vi "Framework Configuration.Get All Transfer Configurations.vi"(8 "error in (no error)":errorcluster, 11 "Framework Configuration in":refnum<class "Framework Configuration.lvclass">) -> (0 "error out":errorcluster, 2 "Transfer Configurations":T1[](array[typedef]), 3 "Framework Configuration out":refnum<class "Framework Configuration.lvclass">)   [LabVIEW 2017, in "DSF.Engine.lvlib" / "Framework Configuration.lvclass"]
uses:
  Framework Configuration.lvclass
  DSF Configuration API/1.0.0/Public/Controls/DSF Engine Transfer Configuration.ctl
  DSF Configuration API/1.0.0/Public/Controls/DSF Byte Order.ctl
  DSF Configuration API/1.0.0/Public/Controls/DSF Engine Channel Configuration.ctl
  DSF Configuration API/1.0.0/Public/Controls/DSF Data Type.ctl
  DSF Configuration API/1.0.0/Public/Controls/DSF Settings Info.ctl
  Framework Configuration.lvclass/Framework Configuration.ctl
  DSF Configuration API/1.0.0/DSF Configuration API.lvlib
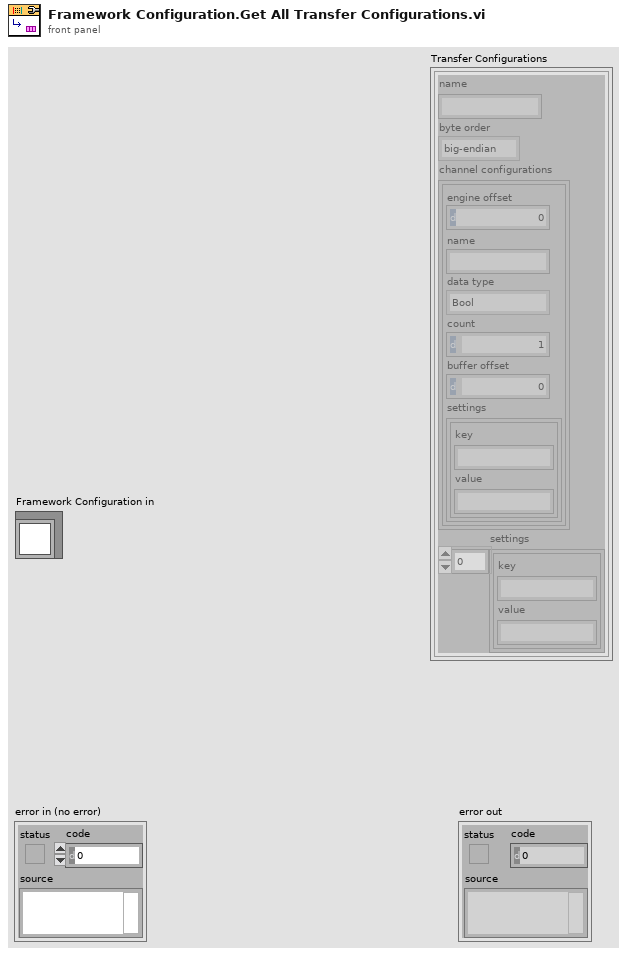
[diagram p1: front panel]
types:
  T1 = typedef "DSF Configuration API.lvlib/DSF Engine Transfer Configuration.ctl" = cluster{"name":string, "byte order":T2, "channel configurations":T3[], "settings":T5}
  T2 = typedef "DSF Configuration API.lvlib/DSF Byte Order.ctl" = enum8{"big-endian", "little-endian"}
  T3 = typedef "DSF Configuration API.lvlib/DSF Engine Channel Configuration.ctl" = cluster{"engine offset":u64, "name":string, "data type":T4, "count":u64, "buffer offset":u64, "settings":T5}
  T4 = typedef "DSF Configuration API.lvlib/DSF Data Type.ctl" = enum8{"Bool", "SGL", "DBL", "I8", "I16", "I32", "I64", "U8", "U16", "U32", "U64"}
  T5 = typedef "DSF Configuration API.lvlib/DSF Settings Info.ctl" = cluster{"key":string, "value":string}[]
  T6 = typedef "DSF Configuration API.lvlib/DSF Engine Framework Configuration.ctl" = cluster{"Plugins":T7[]}
  T7 = typedef "DSF Configuration API.lvlib/DSF Engine Plugin Configuration.ctl" = cluster{"name":string, "class":string, "cycle timing":T8, "Transfer Groups":T9[], "settings":T5}
  T8 = typedef "DSF Configuration API.lvlib/DSF Timing Info.ctl" = cluster{"priority":u64, "decimation":u64, "offset":u64}
  T9 = typedef "DSF Configuration API.lvlib/DSF Engine Transfer Group Configuration.ctl" = cluster{"name":string, "direction":T10, "cycle timing":T8, "Transfers":T1[], "settings":T5}
  T10 = typedef "DSF Configuration API.lvlib/DSF Direction.ctl" = enum8{"Tx", "Rx"}
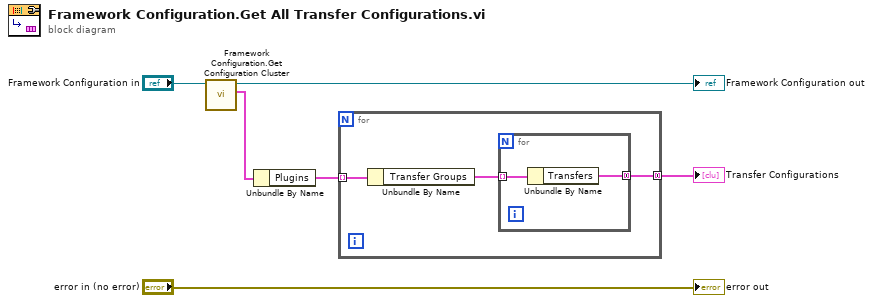
[diagram p0: block diagram]
diagram:
  n1 = call "Framework Configuration.Get Configuration Cluster.vi"("Framework Configuration in"="Framework Configuration in") -> ("Framework Configuration"=w1:T6, "Framework Configuration out"=→"Framework Configuration out":refnum<class "Framework Configuration.lvclass">)  [unwired: 9 in]
  n2 = Unbundle By Name(w1) -> ("Plugins"=w5:T7[])
  n3 = for {
    tunnel: w5 -> [w9] mode=indexing
    tunnel: [w7] -> w4 mode=concatenating
    n4 = Unbundle By Name(w9) -> ("Transfer Groups"=w8:T9[])
    n5 = for {
      tunnel: w8 -> [w11] mode=indexing
      tunnel: [w10] -> w7 mode=concatenating
      n6 = Unbundle By Name(w11) -> ("Transfers"=w10:T1[])
    }
  }
  "Transfer Configurations" <- w4
  "error out" <- "error in (no error)"
